vi "intensity_cursorHandler.vi"(4 "End":dbl, 6 "Start":dbl, 9 "Min":dbl, 10 "Max":dbl) -> ()   [LabVIEW 2019]
uses:
  REFS.vi
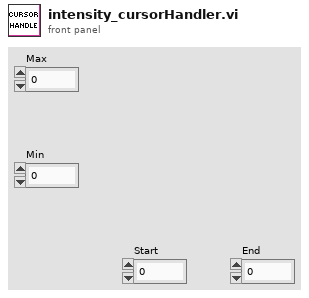
[diagram p1: front panel]
types:
  T1 = cluster{string, i32, i32, i32, bool, bool, i32, i32, i32, cluster{"Numeric":dbl, dbl}, i32, i32, i32[], bool, i32, cluster{dbl, dbl}}
  T2 = cluster{string, i32, i32, i32, bool, bool, i32, i32, i32, cluster{"Numeric":dbl, dbl}, i32, i32, i32[], bool, i32, cluster{dbl, dbl}}[]
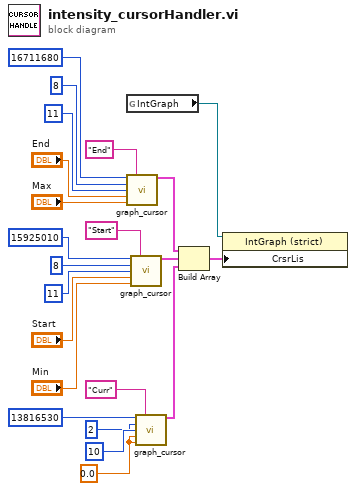
[diagram p0: block diagram]
diagram:
  w20 = 0.0 ("Y")
  n1 = global read "REFS.vi" "IntGraph"() -> (w1:refnum<vi>)
  n2 = call "graph_cursor.vi"("Colour"=16711680, "Name"="End", "Style"=8, "Point style"=11, "X"="End", "Y"="Max") -> ("Cursor Cluster"=w10:T1)  [unwired: 9 in]
  n3 = call "graph_cursor.vi"("Colour"=15925010, "Name"="Start", "Style"=8, "Point style"=11, "X"="Start", "Y"="Min") -> ("Cursor Cluster"=w11:T1)  [unwired: 9 in]
  n4 = call "graph_cursor.vi"("Colour"=13816530, "Name"="Curr", "Style"=2, "Point style"=10, "X"=w20, "Y"=w20) -> ("Cursor Cluster"=w15:T1)  [unwired: 9 in]
  n5 = Build Array(w10, w11, w15) -> (w12:T2)
  n6 = property on="Property Node" class="IntGraph (strict)"(reference=w1, "CrsrLis"=w12) -> ()  [unwired: 1 in, 2 out]
